vi "ExEMCircBufROInframeSeq.vi"() -> ()   [LabVIEW 2010]
uses:
  CamHandle.vi
panel:
  in  "Number of images":u32=25
  in  "OK Button":bool
  out "Collecting":bool
  in  "av gain":dbl format="%.2f"
  in  "Invert Logic output":bool
  in  "Logic Output":i32
  in  "Fan":i32=1
  in  "ADC Gain":u32
  out "ADC Speed (Khz)":u32
  in  "Fast ADC":bool
  in  "X Start":u32=1 min=1 step=1
  in  "Y Bin":u32=1 min=1 step=1
  in  "X End":u32=512 min=1 max=512 step=1
  in  "X Bin":u32=1 min=1 step=1
  in  "Y Start":u32=1 min=1 step=1
  in  "Y End":u32=512 min=1 max=512 step=1
  in  "Temperature":dbl=-55.0 format="%.2f"
  in  "Exposure":dbl min=0.0 step=0.001 format="%.3f"
  out "error out":errorcluster
  in  "error in (no error)":errorcluster
  # "ExEMCircBufROInframeSeq:\nThis example allows a single ROI\nto be programmed up. It then runs\nin sync (nframe mode displaying \nthe ROI data as it comes in.\nNote: this example requires the \ncamera support circular buffers.\nThis example also shows how to \nsetup the cascade to run in over-\nlapped mode and how to set the\non-chip multiplication gain and how\nto set the readout port."
  # "Warning: you must open and run once the VI ExOpenGlobalCam.vi.\nYou only need to run it once then you can run this Example VI as many\ntimes as you want."
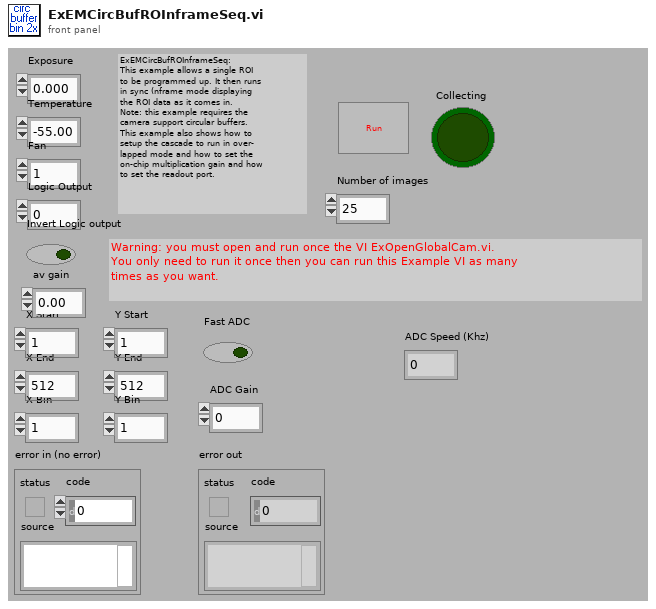
[diagram p1: front panel]
types:
  T1 = cluster{"X Start":u32, "X End":u32, "X Bin":u32, "Y Start":u32, "Y End":u32, "Y Bin":u32}
  T2 = cluster{"acquire focus mode":u32, "Exposure":dbl, "Number of images":u32, "Software accumulation":u32}
  T3 = cluster{"Camera Handle":u32, "File Handle":u32, "Display Handle":u32, "Image Handle":u32}
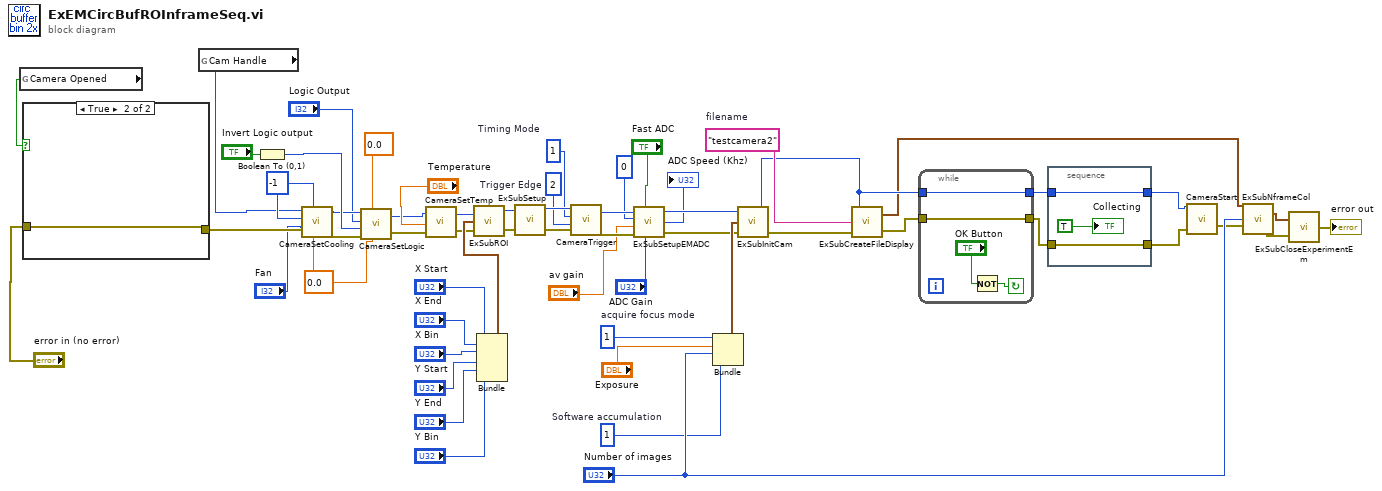
[diagram p0: block diagram]
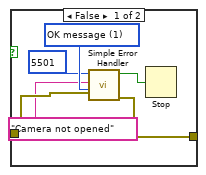
[diagram p2: hidden frame]
diagram:
  w15 = 0.0
  w16 = -1
  w48 = u32 1  # Timing Mode
  w49 = u32 2  # Trigger Edge
  w52 = u32 1  # acquire focus mode
  w50 = u32 1  # Software accumulation
  w58 = "testcamera2"  # filename
  n1 = global read "CamHandle.vi" "Camera Opened"() -> (w25:bool)
  n2 = case shown="True" w25 {
    tunnel: "error in (no error)" -> [w63 w65]
    tunnel: [w62 w65] -> w23
    frame False {
      w64 = u16 1 items=["no dialog", "OK message", "continue or stop message"] ("type of dialog (OK msg:1)")
      n3 = call <vilib>:"Simple Error Handler.vi"("error code (no error:0)"=5501, "error source (\" \")"="Camera not opened", "type of dialog (OK msg:1)"=w64, "error in (no error)"=w63) -> ("error?"=w60:bool, "error out"=w62:errorcluster)  [unwired: 1 in, 3 out]
      n4 = Stop(stop? (T)=w60) -> ()
    }
    frame True {
    }
  }
  n5 = global read "CamHandle.vi" "Cam Handle"() -> (w11:u32)
  n6 = Boolean To (0,1)(Boolean="Invert Logic output") -> (0, 1=w19:i16)
  n7 = call <userlib>:"CameraSetCooling.vi"("Reserved"=w15, "Cooling Mode"=w16, "error in (no error)"=w23, "Fan"="Fan", "Cooling"=w16, "Camera Handle"=w11) -> ("error out"=w22:errorcluster, "Camera Handle"=w18:u32)
  n8 = call <userlib>:"CameraSetLogic.vi"("Reserved 2"=w15, "Reserved"=0.0, "error in (no error)"=w22, "Invert Logic"=w19, "Logic Output"="Logic Output", "Camera Handle"=w18) -> ("error out"=w21:errorcluster, "Camera Handle"=w14:u32)
  n9 = call <userlib>:"CameraSetTemp.vi"("error in (no error)"=w21, "Temperature"="Temperature", "Camera Handle"=w14) -> ("error out"=w39:errorcluster, "Camera Handle"=w38:u32)
  n10 = Bundle("X Start"="X Start", "X End"="X End", "X Bin"="X Bin", "Y Start"="Y Start", "Y End"="Y End", "Y Bin"="Y Bin") -> (w41:T1)  [unwired: 1 in]
  n11 = call "ExSubROI.vi"("error in (no error)"=w39, "ROI"=w41, "Camera Handle"=w38) -> ("error out"=w36:errorcluster, "Camera Handle"=w40:u32)
  n12 = call "ExSubSetup.vi"("error in (no error)"=w36, "Camera Handle"=w40) -> ("error out"=w35:errorcluster, "Camera Handle"=w53:u32)
  n13 = call <userlib>:"CameraTrigger.vi"("error in"=w35, "Trigger Edge"=w49, "Timing Mode"=w48, "Camera Handle"=w53) -> ("error out"=w33:errorcluster, "Camera Handle"=w34:u32)
  n14 = call "ExSubSetupEMADC.vi"("Camera Handle"=w34, "Fast ADC"="Fast ADC", "ReadOut Port"=0, "Avalanche Gain\nOnly valid for \nport 0"="av gain", "ADC Gain"="ADC Gain", "error in (no error)"=w33) -> ("Camera Handle"=w31:u32, "ADC Speed (Khz)"=→"ADC Speed (Khz)":u32, "error out"=w32:errorcluster)
  n15 = Bundle("acquire focus mode"=w52, "Exposure"="Exposure", "Number of images"="Number of images", "Software accumulation"=w50) -> (w56:T2)  [unwired: 1 in]
  n16 = call "ExSubInitCam.vi"("error in (no error)"=w32, "Camera Information"=w56, "Camera Handle"=w31) -> ("error out"=w55:errorcluster, "Camera Handle"=w7:u32)
  n17 = call "ExSubCreateFileDisplay.vi"("error in (no error)"=w55, "File and Display Name"=w58, "Camera Handle"=w7) -> ("error out"=w4:errorcluster, "Handles Out"=w1:T3)
  n18 = while {
    tunnel: w7 -> [w67]
    tunnel: [w67] -> w6
    tunnel: w4 -> [w66]
    tunnel: [w66] -> w3
    stop <- w69 continue-if-true
    n19 = Not(x="OK Button") -> (.not. x?=w69:bool)
  }
  n20 = stacked-sequence {
    tunnel: w6 -> [w71]
    tunnel: [w71] -> w5
    tunnel: w3 -> [w70]
    tunnel: [w70] -> w2
    frame #0 {
      "Collecting" <- TRUE
    }
  }
  n21 = call <userlib>:"CameraStart.vi"("error in"=w2, "Camera Handle"=w5) -> ("error out"=w10:errorcluster)  [unwired: 1 out]
  n22 = call "ExSubNframeCol.vi"("error in (no error)"=w10, "Number of Images"="Number of images", "Handle Cluster"=w1) -> ("error out"=w9:errorcluster, "Handle Cluster"=w8:T3)
  n23 = call "ExSubCloseExperimentEm.vi"("error in (no error)"=w9, "Handles In"=w8) -> ("error out"=→"error out":errorcluster)
